vi "MListbox SelMode.vi"(8 "错误输入":errorcluster, 11 "Mlistbox Ref":refnum<vi>) -> (0 "错误输出":errorcluster, 1 "Array?":bool, 2 "SelMode":T1, 3 "Mlistbox Ref Dup":refnum<vi>)   [LabVIEW 2012, in "Mlistbox Tools.lvlib"]
uses:
  Mlistbox Tools.lvlib
  ListBox/Custom Type/SelMode.ctl
  ListBox/Listbox Tool.lvlib
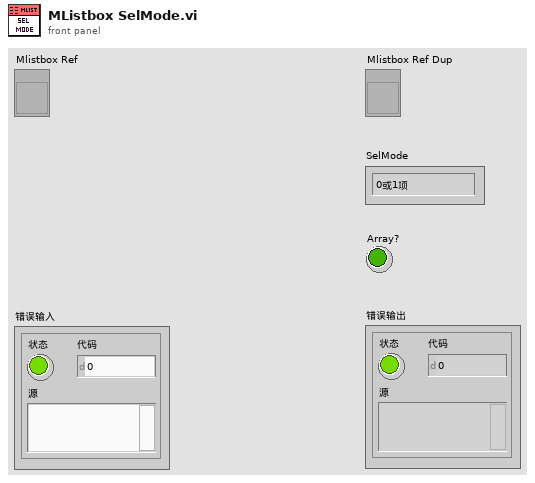
[diagram p1: front panel]
types:
  T1 = typedef "Listbox Tool.lvlib/SelMode.ctl" = enum16{"0或1项", "1项", "0或多项", "1或多项"}
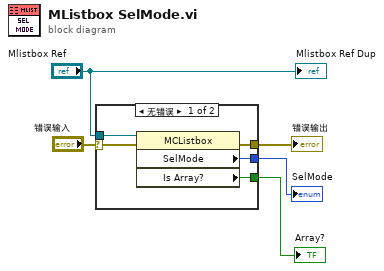
[diagram p0: block diagram]
diagram:
  n1 = case shown="无错误" "错误输入" {
    selector: "错误输入" -> [w9 w11]
    tunnel: [w7 w11] -> w4
    tunnel: "Mlistbox Ref" -> [w10 _]
    tunnel: [w8 _] -> w2
    tunnel: [w6 _] -> w1
    frame No Error {
      n2 = property class="MCListbox"(reference=w10, error in=w9) -> (error out=w7:errorcluster, "SelMode"=w8:i32, "Is Array?"=w6:bool)  [unwired: 1 out]
    }
    frame Error {
    }
  }
  "错误输出" <- w4
  "SelMode" <- w2
  "Array?" <- w1
  "Mlistbox Ref Dup" <- "Mlistbox Ref"
